vi "Timed One-Shot (SubVI).vi"(0 "ENABLE OUTPUT":bool, 7 "Time Setpoint [s]":dbl=10.0, 11 "START/RESET":bool) -> (4 "Output":bool, 8 "Elapsed Time [s]":dbl format="%.1f")   [LabVIEW 2012]
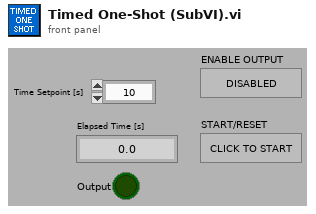
[diagram p1: front panel]
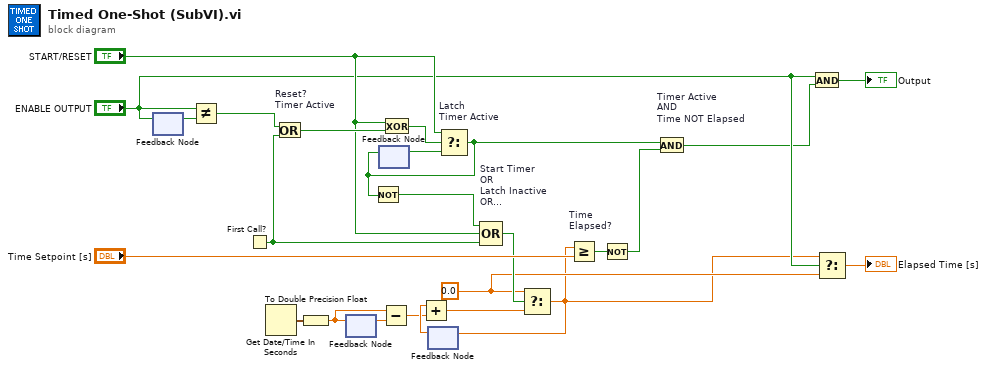
[diagram p0: block diagram]
diagram:
  w5 = 0.0 ("t")
  n1 = feedback #1() -> (w21:bool)  [unwired: 1 in]
  n2 = feedback-in #1("ENABLE OUTPUT") -> ()
  n3 = Not Equal?(x="ENABLE OUTPUT", y=w21) -> (x != y?=w7:bool)
  n4 = First Call?() -> (First Call?: T/F=w12:bool)
  n5 = Get Date/Time In Seconds() -> (seconds since 1Jan1904=w18:timestamp)
  n6 = Or "Reset?\nTimer Active"(x=w7, y=w12) -> (x .or. y?=w24:bool)
  n7 = To Double Precision Float(number=w18) -> (double precision float=w17:dbl)
  n8 = feedback #2() -> (w19:dbl)  [unwired: 1 in]
  n9 = feedback-in #2(w17) -> ()
  n10 = feedback #3() -> (w23:bool)  [unwired: 1 in]
  n11 = Subtract(x=w17, y=w19) -> (x-y=w16:dbl)
  n12 = Exclusive Or(1:w24, 2:"START/RESET") -> (0:w22:bool)
  n13 = feedback #4() -> (w20:dbl)  [unwired: 1 in]
  n14 = Add(x=w20, y=w16) -> (x+y=w15:dbl)
  n15 = Select "Latch\nTimer Active"(t="START/RESET", s=w22, f=w23) -> (s? t:f=w10:bool)
  n16 = Not(x=w10) -> (.not. x?=w9:bool)
  n17 = feedback-in #3(w10) -> ()
  n18 = Compound Arithmetic op=OR "Start Timer\nOR\nLatch Inactive\nOR\nFirst Call"(w9, "START/RESET", w12) -> (w11:bool)
  n19 = Select(t=w5, s=w11, f=w15) -> (s? t:f=w2:dbl)
  n20 = feedback-in #4(w2) -> ()
  n21 = Greater Or Equal? "Time\nElapsed?"(x=w2, y="Time Setpoint [s]") -> (x >= y?=w13:bool)
  n22 = Not(x=w13) -> (.not. x?=w14:bool)
  n23 = And "Timer Active\nAND\nTime NOT Elapsed"(x=w10, y=w14) -> (x .and. y?=w4:bool)
  n24 = And(x="ENABLE OUTPUT", y=w4) -> (x .and. y?=→"Output":bool)
  n25 = Select(t=w2, s="ENABLE OUTPUT", f=w5) -> (s? t:f=→"Elapsed Time [s]":dbl)
